vi "Main.vi"() -> ()   [LabVIEW 2018]
panel:
  in  "Oven IP address":string
  out "Oven state":bool
  out "Reflow uptime":dbl
  in  "Set temperature":dbl
  out "Waveform Chart":dbl(graph)
  out "Heater state":bool
  in  "Enable/Disable":bool
  out "Current temperature:":dbl
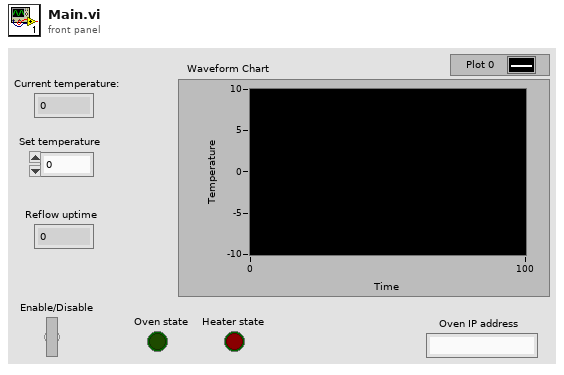
[diagram p1: front panel]
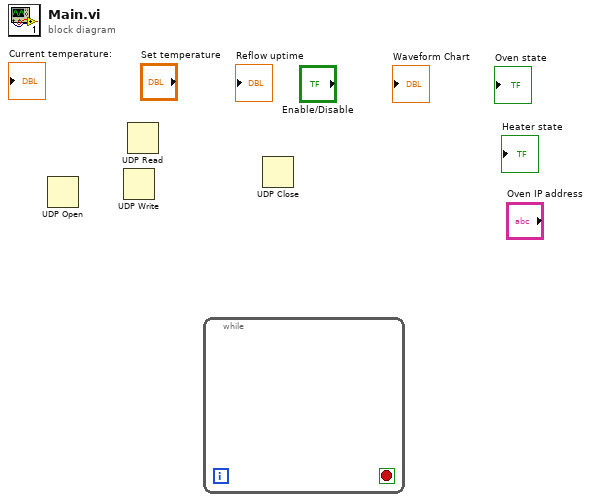
[diagram p0: block diagram]
diagram:
  n1 = UDP Open() -> ()  [unwired: 5 in, 3 out]
  n2 = UDP Write() -> ()  [unwired: 6 in, 2 out]
  n3 = UDP Read() -> ()  [unwired: 4 in, 5 out]
  n4 = while {
    stop <- _ stop-if-true
  }
  n5 = UDP Close() -> ()  [unwired: 2 in, 2 out]
